vi "Encoder Calculus Motor 2.vi"(8 "Velocity Interval (uSec)":i32, 11 "Position (Counts)":i16) -> (1 "Speed Output":T4, 2 "Position Output":T3)   [LabVIEW 2013]
panel:
  in  "Values":T1
  out "output cluster":T2
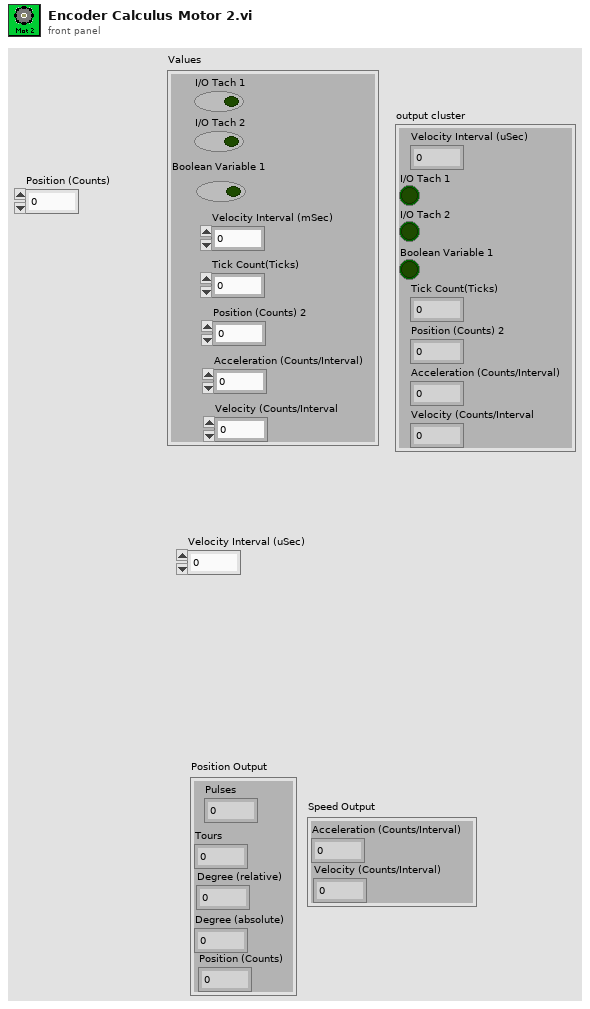
[diagram p1: front panel]
types:
  T1 = cluster{"Velocity Interval (mSec)":i32, "I/O Tach 1":bool, "I/O Tach 2":bool, "Boolean Variable 1":bool, "Tick Count(Ticks)":u32, "Position (Counts) 2":i16, "Acceleration (Counts/Interval)":i16, "Velocity (Counts/Interval":i16}
  T2 = cluster{"Velocity Interval (uSec)":i32, "I/O Tach 1":bool, "I/O Tach 2":bool, "Boolean Variable 1":bool, "Tick Count(Ticks)":u32, "Position (Counts) 2":i16, "Acceleration (Counts/Interval)":i16, "Velocity (Counts/Interval":i16}
  T3 = cluster{"Pulses":i32, "Degree (absolute)":i32, "Degree (relative)":i32, "Tours":i32, "Position (Counts)":i32}
  T4 = cluster{"Velocity (Counts/Interval)":i32, "Acceleration (Counts/Interval)":i32}
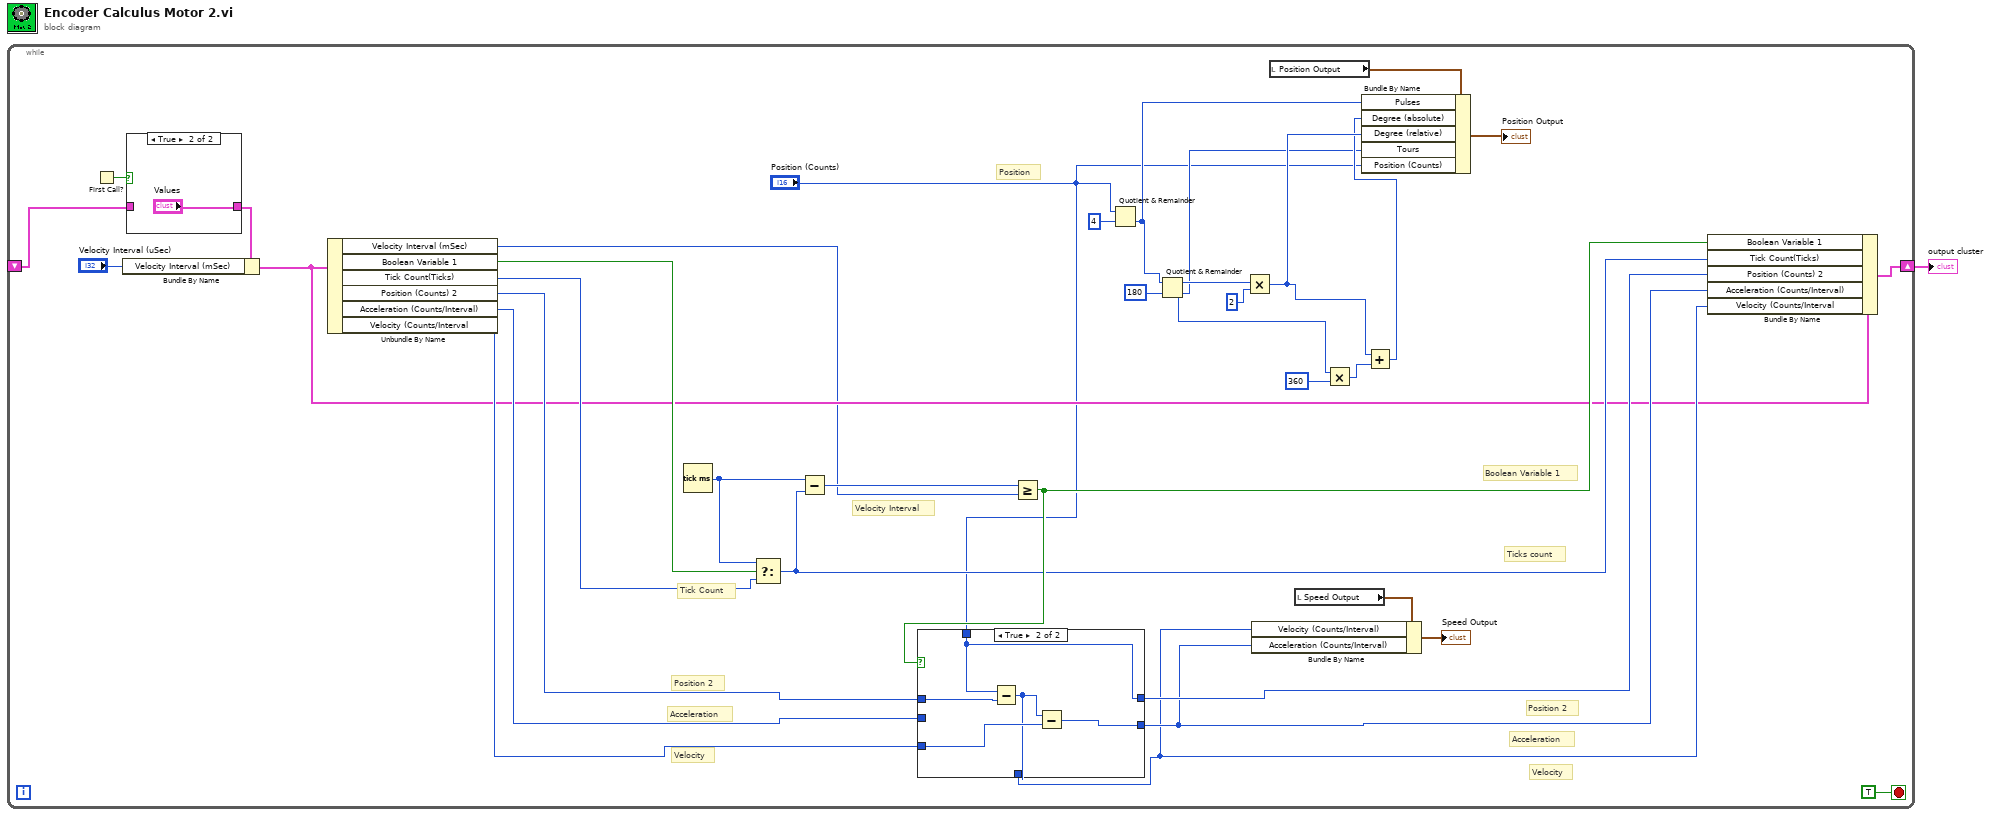
[diagram p0: block diagram]
diagram:
  n1 = while {
    shift-right: [w11] -> w1
    shift-left: _ -> [w6]
    stop <- TRUE stop-if-true
    # "Velocity Interval"
    # "Tick Count"
    # "Position 2"
    # "Acceleration"
    # "Velocity"
    # "Position"
    # "Boolean Variable 1"
    # "Ticks count"
    # "Position 2"
    # "Acceleration"
    # "Velocity"
    n2 = First Call?() -> (First Call?: T/F=w8:bool)
    n3 = case shown="True" w8 {
      tunnel: [w37 "Values"] -> w7
      tunnel: w6 -> [w37 _]
      frame False {
      }
      frame True {
      }
    }
    n4 = Bundle By Name(cluster=w7, "Velocity Interval (mSec)"="Velocity Interval (uSec)") -> (w5:T1)
    n5 = Unbundle By Name(w5) -> ("Velocity Interval (mSec)"=w3:i32, "Boolean Variable 1"=w21:bool, "Tick Count(Ticks)"=w20:u32, "Position (Counts) 2"=w17:i16, "Acceleration (Counts/Interval)"=w18:i16, "Velocity (Counts/Interval"=w19:i16)
    n6 = Tick Count (ms)() -> (millisecond timer value=w2:u32)
    n7 = Select(t=w2, s=w21, f=w20) -> (s? t:f=w15:u32)
    n8 = Subtract(x=w2, y=w15) -> (x-y=w36:u32)
    n9 = Greater Or Equal?(x=w36, y=w3) -> (x >= y?=w16:bool)
    n10 = case shown="True" w16 {
      tunnel: w17 -> [w41 w46]
      tunnel: "Position (Counts)" -> [_ w45]
      tunnel: [w41 w45] -> w14
      tunnel: [w40 w44] -> w13
      tunnel: w19 -> [w39 w43]
      tunnel: [w39 w42] -> w12
      tunnel: w18 -> [w40 _]
      frame False {
      }
      frame True {
        n11 = Subtract(x=w45, y=w46) -> (x-y=w42:i16)
        n12 = Subtract(x=w42, y=w43) -> (x-y=w44:i16)
      }
    }
    n13 = Quotient & Remainder(x="Position (Counts)", y=i16 4) -> (floor(x/y)=w29:i16)  [unwired: 1 out]
    n14 = Quotient & Remainder(x=w29, y=i16 180) -> (x-y*floor(x/y)=w34:i16, floor(x/y)=w26:i16)
    n15 = Multiply(x=w34, y=i16 2) -> (x*y=w28:i16)
    n16 = local read "Position Output"() -> (w24:T3)
    n17 = local read "Speed Output"() -> (w23:T4)
    n18 = Bundle By Name(cluster=w23, "Velocity (Counts/Interval)"=w12, "Acceleration (Counts/Interval)"=w13) -> (→"Speed Output":T4)
    n19 = Multiply(x=w26, y=i16 360) -> (x*y=w31:i16)
    n20 = Add(x=w28, y=w31) -> (x+y=w27:i16)
    n21 = Bundle By Name(cluster=w24, "Pulses"=w29, "Degree (absolute)"=w27, "Degree (relative)"=w28, "Tours"=w26, "Position (Counts)"="Position (Counts)") -> (→"Position Output":T3)
    n22 = Bundle By Name(cluster=w5, "Boolean Variable 1"=w16, "Tick Count(Ticks)"=w15, "Position (Counts) 2"=w14, "Acceleration (Counts/Interval)"=w13, "Velocity (Counts/Interval"=w12) -> (w11:T1)
  }
  "output cluster" <- w1
